vi "SaveFrontPanel.vi"(10 "path to PNG file":path, 11 "vi path":path) -> ()   [LabVIEW 2013]
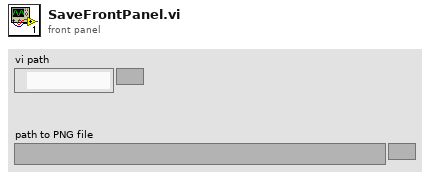
[diagram p1: front panel]
types:
  T1 = typedef "imagedata.ctl" = cluster{"image type":i32, "image depth":i32, "image":u8[], "mask":u8[], "colors":u32[], "Rectangle":cluster{"left":i16, "top":i16, "right":i16, "bottom":i16}}
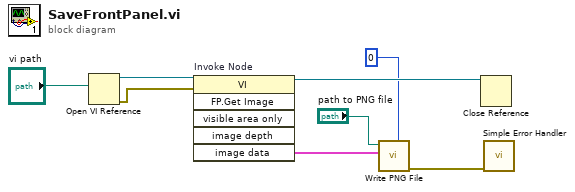
[diagram p0: block diagram]
diagram:
  n1 = Open VI Reference(vi path="vi path") -> (vi reference=w8:refnum<vi>, error out=w7:errorcluster)  [unwired: 5 in]
  n2 = invoke on="Invoke Node" class="VI" method="FP.Get Image"(reference=w8, error in=w7) -> (reference out=w3:refnum<vi>, "image data"=w6:T1)  [unwired: 4 in, 4 out]
  n3 = call <vilib>:"Write PNG File.vi"("compression (default)"=0, "image data"=w6, "path to PNG file"="path to PNG file") -> ("error out"=w4:errorcluster)  [unwired: 7 in, 1 out]
  n4 = Close Reference(reference=w3) -> ()  [unwired: 1 in, 1 out]
  n5 = call <vilib>:"Simple Error Handler.vi"("error in (no error)"=w4) -> ()  [unwired: 4 in, 5 out]
